vi "analyseData.vi"(8 "error in (no error)":errorcluster, 10 "HGF_VariantDataObject in":refnum<class "HGF_VariantDataObject.lvclass">, 11 "Wfm_Amplitude in":refnum<class "Wfm_Amplitude.lvclass">) -> (0 "error out":errorcluster, 2 "HGF_VariantDataObject out":refnum<class "HGF_VariantDataObject.lvclass">, 3 "Wfm_Amplitude out":refnum<class "Wfm_Amplitude.lvclass">)   [LabVIEW 2012, in "MyApp.lvlib" / "Wfm_Amplitude.lvclass"]
doc: "Analyse data contained in HGF_DataVariantObject by using the HGF_DataAnalysator objects and optionally compining their results for a summaray result.\n\nThis is a dynamic dispatch VI to be overwritten by child classes."
uses:
  Wfm_Amplitude.lvclass
  HGF_LVC/HGF_BaseClasses/HGF_VariantDataObject/HGF_VariantDataObject.lvclass
  Wfm_Amplitude.lvclass/Wfm_Amplitude.ctl
  <vilib>/measure/mascope.llb/Amplitude and Levels 1 chan.vi
  <vilib>/measure/NI_MAPro.lvlib
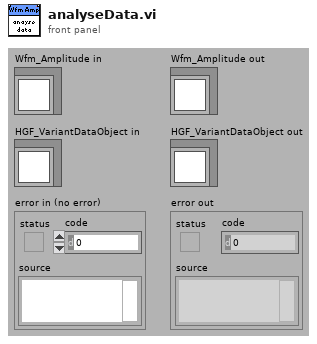
[diagram p1: front panel]
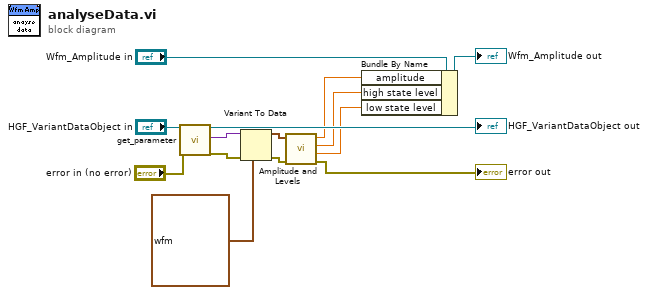
[diagram p0: block diagram]
diagram:
  n1 = call "get_parameter.vi"("HGF_VariantDataObject"="HGF_VariantDataObject in", "error in (no error)"="error in (no error)") -> ("dup HGF_VariantDataObject"=→"HGF_VariantDataObject out":refnum<class "HGF_VariantDataObject.lvclass">, "parameter"=w12:variant, "error out"=w9:errorcluster)  [unwired: 14 in, 1 out]
  n2 = Variant To Data(error in=w9, type=waveform(dbl) {"t0"=timestamp(0 s since 1904-01-01), "dt"=0.0, "Y"=[]} ("signal in"), Variant=w12) -> (data=w6:waveform(dbl), error out=w5:errorcluster)
  n3 = call-poly <vilib>:"Amplitude and Levels.vi"("error in (no error)"=w5, "signal in"=w6) -> ("error out"=→"error out":errorcluster, "low state level"=w2:dbl, "high state level"=w3:dbl, "amplitude"=w4:dbl)  [unwired: 6 in]
  n4 = Bundle By Name(cluster="Wfm_Amplitude in", "amplitude"=w4, "high state level"=w3, "low state level"=w2) -> (→"Wfm_Amplitude out":refnum<class "Wfm_Amplitude.lvclass">)
